vi "Robot Command.vi"(9 "Array In":u8[](array[numeric]), 11 "Robot":T1={"id"=0, "function"=enum."Attacker", "x"=0.0, "y"=0.0, "orientation"=0.0, "v_tangent"=0.0, "v_normal"=0.0, "v_ang"=0.0, "kick_x"=0.0, "kick_z"=0.0, "dribble"=FALSE, "Timestamp"=timestamp(0 s since 1904-01-01), "estimatives"={"est_v_tangent"=0.0, "est_v_normal"=0.0, "est_vx"=0.0, "est_vy"=0.0, "Pos Robot Est"=[]}, "dest_x_kick"=0.0, "dest_y_kick"=0.0, "Gap Coord"=[], "States"=enum."GoToTangent", "Path "=[], "Path  Smooth"=[], "Dest"=[]}) -> (1 "Array":u8[](array[numeric]))   [LabVIEW 2017]
uses:
  Core/AI Robot.ctl
  Intel/Functions Enum.ctl
  Intel/AttackerStates.ctl
  Path Planning/RRT/PathDests.ctl
  Path Planning/RRT/PathDest.ctl
  Varint Encoder uint32.vi
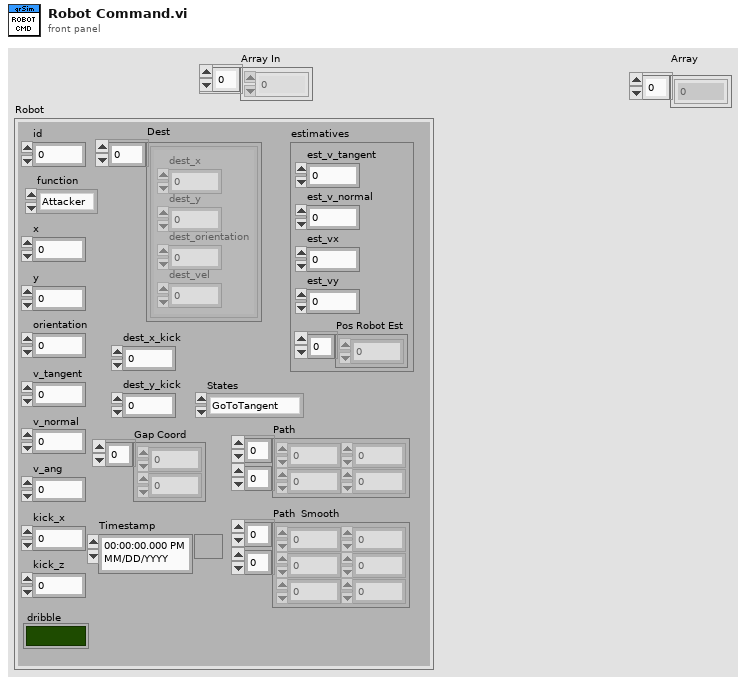
[diagram p1: front panel]
types:
  T1 = typedef "AI Robot.ctl" = cluster{"id":u32, "function":T2, "x":dbl, "y":dbl, "orientation":dbl, "v_tangent":dbl, "v_normal":dbl, "v_ang":dbl, "kick_x":dbl, "kick_z":dbl, "dribble":bool, "Timestamp":timestamp, "estimatives":cluster{"est_v_tangent":dbl, "est_v_normal":dbl, "est_vx":dbl, "est_vy":dbl, "Pos Robot Est":dbl[]}, "dest_x_kick":dbl, "dest_y_kick":dbl, "Gap Coord":dbl[], "States":T3, "Path ":dbl[][], "Path  Smooth":dbl[][], "Dest":T4}
  T2 = typedef "Functions Enum.ctl" = enum16{"Attacker", "Goalie", "Defender", "Striker", "Goto 0", "Dummy", "Kicker", "ZigZag"}
  T3 = typedef "AttackerStates.ctl" = enum16{"Pass", "GoToTangent", "BallGetting", "GoToKick", "Rotate anti-clockwise", "Rotate Clockwise", ""}
  T4 = typedef "PathDests.ctl" = T5[]
  T5 = typedef "PathDest.ctl" = cluster{"dest_x":dbl, "dest_y":dbl, "dest_orientation":dbl, "dest_vel":dbl}
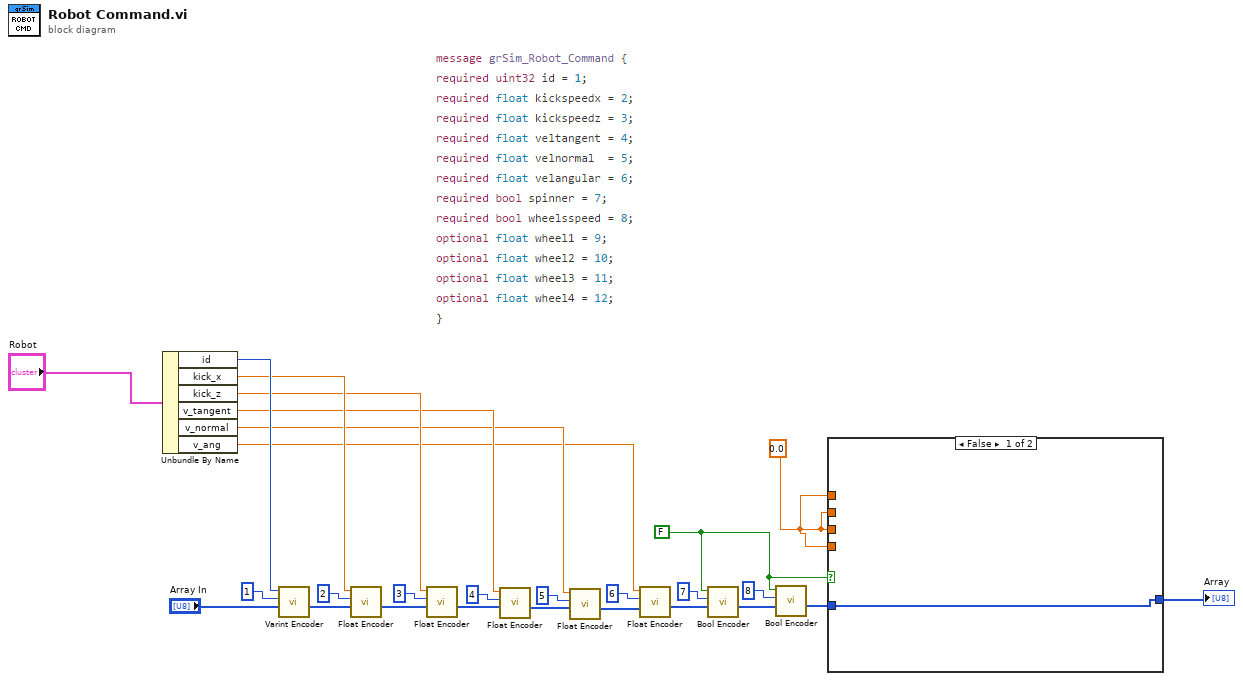
[diagram p0: block diagram]
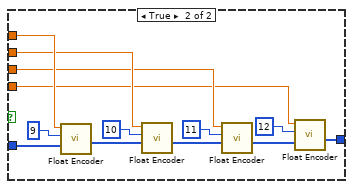
[diagram p2: hidden frame]
diagram:
  w1 = 0.0
  w2 = FALSE
  n1 = Unbundle By Name("Robot") -> ("id"=w27:u32, "kick_x"=w22:dbl, "kick_z"=w13:dbl, "v_tangent"=w12:dbl, "v_normal"=w11:dbl, "v_ang"=w10:dbl)
  n2 = call-poly "Varint Encoder.vi"("Array In"="Array In", "Key"=u32 1, "Value"=w27) -> ("Array"=w24:u8[])  [unwired: 8 in]
  n3 = call "Float Encoder.vi"("Array In"=w24, "Key"=u32 2, "Value"=w22) -> ("Array"=w17:u8[])  [unwired: 8 in]
  n4 = call "Float Encoder.vi"("Array In"=w17, "Key"=u32 3, "Value"=w13) -> ("Array"=w16:u8[])  [unwired: 8 in]
  n5 = call "Float Encoder.vi"("Array In"=w16, "Key"=u32 4, "Value"=w12) -> ("Array"=w15:u8[])  [unwired: 8 in]
  n6 = call "Float Encoder.vi"("Array In"=w15, "Key"=u32 5, "Value"=w11) -> ("Array"=w14:u8[])  [unwired: 8 in]
  n7 = call "Float Encoder.vi"("Array In"=w14, "Key"=u32 6, "Value"=w10) -> ("Array"=w9:u8[])  [unwired: 8 in]
  n8 = call "Bool Encoder.vi"("Array In"=w9, "Key"=u32 7, "Value"=w2) -> ("Array"=w7:u8[])  [unwired: 8 in]
  n9 = call "Bool Encoder.vi"("Array In"=w7, "Key"=u32 8, "Value"=w2) -> ("Array"=w5:u8[])  [unwired: 8 in]
  n10 = case shown="False" w2 {
    tunnel: w5 -> [w28 w40]
    tunnel: w1 -> [_ w33]
    tunnel: w1 -> [_ w32]
    tunnel: w1 -> [_ w31]
    tunnel: w1 -> [_ w30]
    tunnel: [w28 w29] -> w4
    frame False {
    }
    frame True {
      n11 = call "Float Encoder.vi"("Array In"=w40, "Key"=u32 9, "Value"=w33) -> ("Array"=w36:u8[])  [unwired: 8 in]
      n12 = call "Float Encoder.vi"("Array In"=w36, "Key"=u32 10, "Value"=w32) -> ("Array"=w35:u8[])  [unwired: 8 in]
      n13 = call "Float Encoder.vi"("Array In"=w35, "Key"=u32 11, "Value"=w31) -> ("Array"=w34:u8[])  [unwired: 8 in]
      n14 = call "Float Encoder.vi"("Array In"=w34, "Key"=u32 12, "Value"=w30) -> ("Array"=w29:u8[])  [unwired: 8 in]
    }
  }
  "Array" <- w4
